vi "NI DAQ start.vi"(8 "error in":errorcluster, 11 "DAQmx Device Name":tag="PXI2Slot6") -> (0 "error out":errorcluster, 3 "DAQmx Device Name Out":tag="PXI2Slot6")   [LabVIEW 2020]
uses:
  NI DAQ globals.vi
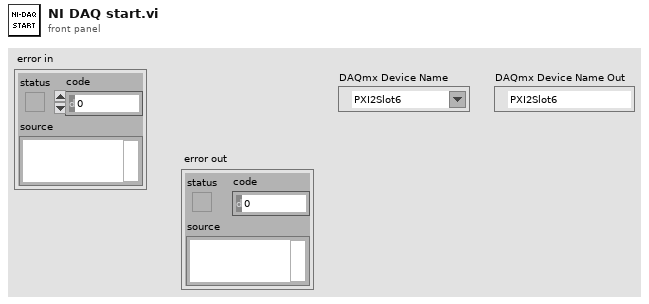
[diagram p1: front panel]
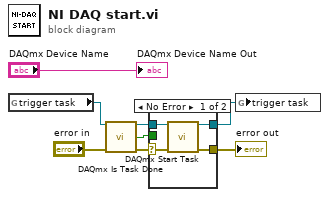
[diagram p0: block diagram]
diagram:
  n1 = global read "NI DAQ globals.vi" "trigger task"() -> (w4:refnum<k21>)
  n2 = call <vilib>:"DAQmx Is Task Done.vi"("task/channels in"=w4, "error in"="error in") -> ("task out"=w7:refnum<k21>, "task done?"=w6:bool, "error out"=w5:errorcluster)  [unwired: 11 in]
  n3 = case shown="No Error" w5 {
    selector: w5 -> [w10 w14]
    tunnel: [w12 w14] -> w1
    tunnel: w6 -> [_ _]
    tunnel: w7 -> [w11 w13]
    tunnel: [w9 w13] -> w3
    frame No Error {
      n4 = call <vilib>:"DAQmx Start Task.vi"("task/channels in"=w11, "error in"=w10) -> ("task out"=w9:refnum<k21>, "error out"=w12:errorcluster)  [unwired: 12 in]
    }
    frame Error {
    }
  }
  "error out" <- w1
  n5 = global write "NI DAQ globals.vi" "trigger task"(w3) -> ()
  "DAQmx Device Name Out" <- "DAQmx Device Name"
